vi "Stop Measurements.vi"(6 "Controller name":string, 8 "error in (no error)":errorcluster, 10 "Request type":T1, 11 "Monitor Controller in":refnum<class "Monitor Controller.lvclass">) -> (0 "error out":errorcluster, 3 "Monitor Controller out":refnum<class "Monitor Controller.lvclass">)   [LabVIEW 2021, in "Monitor Controller.lvclass"]
uses:
  Monitor Controller.lvclass
  C:/GitHub/LabActor/Worker/Worker Actor.lvclass
  C:/Program Files/National Instruments/LabVIEW 2021/vi.lib/ActorFramework/Actor/Actor.lvclass
  Process Controller/Request type.ctl
  Worker/Worker Actor/Worker Actor.lvclass/Worker Actor.ctl
  <vilib>/ActorFramework/Actor/Actor.lvclass/Actor.ctl
  Update Monitor State Msg/Update Monitor State Msg.lvclass/Update Monitor State Msg.ctl
  <vilib>/ActorFramework/Message Enqueuer/Message Enqueuer.lvclass/Message Enqueuer.ctl
  Template Module/Read State.vi
  <vilib>/ActorFramework/Message Enqueuer/Enqueue.vi
  Update Monitor State Msg/Update Monitor State Msg.lvclass
  C:/Program Files/National Instruments/LabVIEW 2021/vi.lib/ActorFramework/Message/Message.lvclass
  <vilib>/ActorFramework/Message Priority Queue/Priority Enqueue.vi
  Process Controller/Process Controller.lvclass
  <vilib>/ActorFramework/Actor/Actor.lvclass
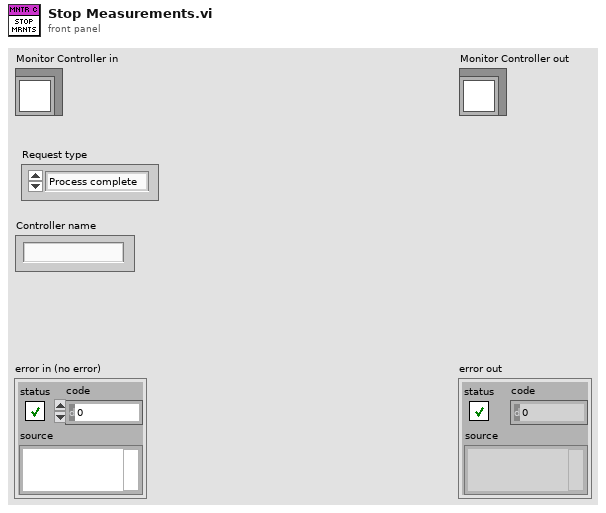
[diagram p1: front panel]
types:
  T1 = typedef "Request type.ctl" = enum16{"Process complete", "User command", "Auto-restart", "Error"}
  T2 = typedef "Worker State.ctl" = enum16{"Idle", "Starting", "Working", "Stopping"}
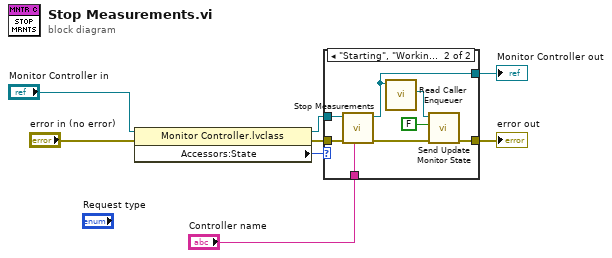
[diagram p0: block diagram]
diagram:
  n1 = property class="Monitor Controller.lvclass"(reference="Monitor Controller in", error in="error in (no error)") -> (reference out=w4:refnum<class "Monitor Controller.lvclass">, error out=w3:errorcluster, "Accessors:State"=w6:T2)
  n2 = case shown="\"Starting\", \"Working\"" w6 {
    tunnel: w3 -> [w9 w18]
    tunnel: w4 -> [w10 w17]
    tunnel: [w10 w12] -> w8
    tunnel: [w9 w16] -> w7
    tunnel: "Controller name" -> [_ w11]
    frame "Idle", Default {
    }
    frame "Starting", "Working" {
      n3 = call-parent "Stop Measurements.vi"("Controller name"=w11, "error in (no error)"=w18, "Measure Controller in"=w17) -> ("error out"=w13:errorcluster, "Measure Controller out"=w12:refnum<class "Monitor Controller.lvclass">)  [unwired: 7 in]
      n4 = call <vilib>:"Read Caller Enqueuer.vi"("Actor"=w12) -> ("Caller Enqueuer"=w15:refnum<class "Message Enqueuer.lvclass">)  [unwired: 10 in]
      n5 = call "Send Update Monitor State.vi"("error in (no error)"=w13, "Monitor Running"=FALSE, "Message Enqueuer"=w15) -> ("error out"=w16:errorcluster)  [unwired: 7 in, 1 out]
    }
  }
  "error out" <- w7
  "Monitor Controller out" <- w8
